vi "Set Exposure Timebase.vi"(8 "error in (no error)":errorcluster, 11 "Camera Quick Settings Panel in":refnum<class "Camera Quick Settings Panel.lvclass">) -> (0 "error out":errorcluster, 3 "Camera Quick Settings Panel out":refnum<class "Camera Quick Settings Panel.lvclass">)   [LabVIEW 2014, in "Camera Quick Settings Panel.lvlib" / "Camera Quick Settings Panel.lvclass"]
uses:
  Camera Quick Settings Panel.lvclass
  Camera Quick Settings Panel.lvclass/Camera Quick Settings Panel.ctl
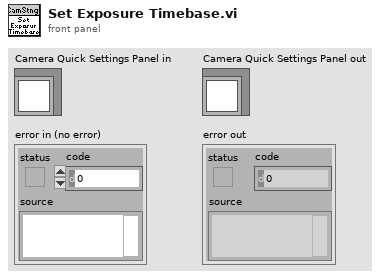
[diagram p1: front panel]
types:
  T1 = cluster{"U32 Value Control":refnum<vi>, "DBL Value Control":refnum<vi>, "String Value Control":refnum<vi>, "Enum Value Control":refnum<vi>, "Boolean Value Control":refnum<vi>, "Command Value Control":refnum<vi>}
  T2 = typedef "IMAQdx.ctl" = refnum<k21>
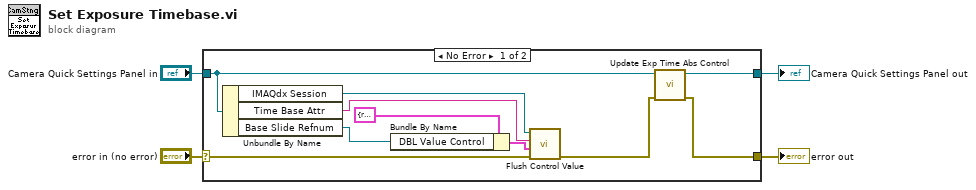
[diagram p0: block diagram]
diagram:
  n1 = case shown="No Error" "error in (no error)" {
    selector: "error in (no error)" -> [w12 w16]
    tunnel: [w5 w16] -> w3
    tunnel: [w7 w15] -> w1
    tunnel: "Camera Quick Settings Panel in" -> [w8 w15]
    frame No Error {
      n2 = Unbundle By Name(w8) -> ("IMAQdx Session"=w13:T2, "Time Base Attr"=w14:string, "Base Slide Refnum"=w9:refnum<vi>)
      n3 = Bundle By Name(cluster=T1 {"U32 Value Control"=refnum, "DBL Value Control"=refnum, "String Value Control"=refnum, "Enum Value Control"=refnum, "Boolean Value Control"=refnum, "Command Value Control"=refnum} ("Tab Control Ref In"), "DBL Value Control"=w9) -> (w10:T1)
      n4 = call "Flush Control Value.vi"("error in (no error)"=w12, "Tab Control Ref In"=w10, "ActiveAttribute"=w14, "Session In"=w13) -> ("error out"=w6:errorcluster)  [unwired: 2 in, 1 out]
      n5 = call-dynamic "Update Exp Time Abs Control.vi"("error in (no error)"=w6, "Camera Quick Settings Panel in"=w8) -> ("error out"=w5:errorcluster, "Camera Quick Settings Panel out"=w7:refnum<class "Camera Quick Settings Panel.lvclass">)  [unwired: 8 in]
    }
    frame Error {
    }
  }
  "error out" <- w3
  "Camera Quick Settings Panel out" <- w1
